vi "OA Initialize.vi"(8 "error in (no error)":errorcluster, 10 "uiFileNameLen":u32, 11 "pcFilename":string) -> (0 "error out":errorcluster, 3 "function return":u32)   [LabVIEW 2014, in "atmcd32d.lvlib"]
doc: "unsigned int WINAPI OA_Initialize(const char * const pcFilename, unsigned int uiFileNameLen);"
uses:
  atmcd32d.lvlib
  atmcd32d.dll
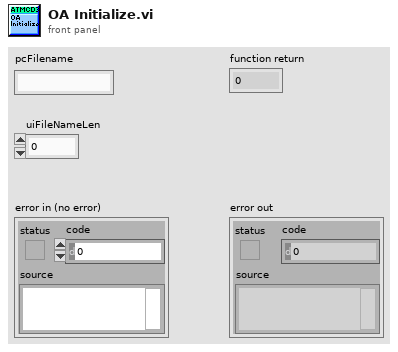
[diagram p1: front panel]
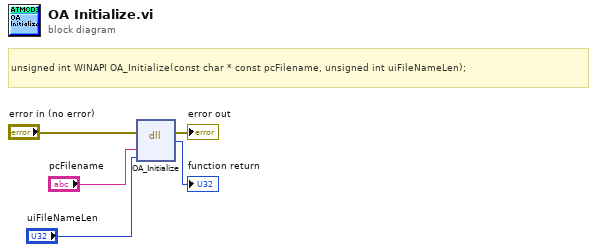
[diagram p0: block diagram]
diagram:
  # "unsigned int WINAPI OA_Initialize(const char * const pcFilename, unsigned int uiFileNameLen);"
  n1 = dll-call lib="C:/Users/Bakir/Documents/Lambda2-Testing/lib/Andorlib/atmcd32d.*" fn="OA_Initialize"(error in="error in (no error)", "pcFilename"="pcFilename", "uiFileNameLen"="uiFileNameLen") -> (error out=→"error out":errorcluster, →"function return":u32)  [unwired: 4 in, 1 out]
